vi "StartMods.vi"(7 "ShowPanel? (f)":bool=TRUE, 8 "ErrorArray":errorcluster[](array[cluster]), 10 "ModuleList":string[](array[string]), 11 "Test.lvclass":refnum<class "Test.lvclass">) -> (0 "ErrorArray":errorcluster[](array[cluster]), 2 "Events":variant[](array[variant]), 3 "Test.lvclass":refnum<class "Test.lvclass">)   [LabVIEW 2018, in "Test.lvclass"]
doc: "This VI instantiates a module..."
uses:
  Test.lvclass
  <userlib>/NIST/ModuleAdminLib/ModuleAdmin/ModuleAdmin.lvclass/ModuleAdmin.ctl
  <userlib>/NIST/ModuleAdminLib/CloneRegistration/CloneRegistration.lvclass
  Test.lvclass/Test.ctl
  <userlib>/NIST/ModuleAdminLib/ModuleAdmin/Accessors/Read CloneRegRef.vi
  Accessors/Write ModuleList.vi
  Accessors/Write ModuleIDs.vi
  Accessors/Write CloneReg.vi
  <vilib>/Utility/error.llb/Error Cluster From Error Code.vi
  <vilib>/ErrorRing/Error Ring.xnode
  <userlib>/NIST/ModuleAdminLib/ModuleAdmin/ModuleAdmin.lvclass
  <userlib>/NIST/NISTErrorLib/NISTErrorLib.lvlib
  Sync/SyncModule/SyncModule.lvlib
  Digitizer/DigitizerModule/DigitizerModule.lvlib
  FGen/FgenModule/FgenModule.lvlib
  Analysis/AnalysisModule/AnalysisModule.lvlib
  Sensor/SensorModule/SensorModule.lvlib
  Scope/ScopeModule/ScopeModule.lvlib
  AcPwr/AcPwrModule/AcPwrModule.lvlib
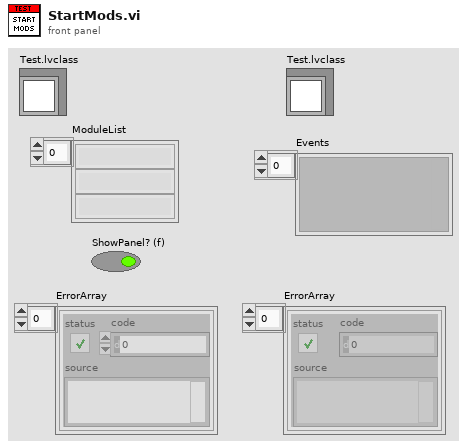
[diagram p1: front panel]
types:
  T1 = typedef "SyncModule.lvlib/clBroadcastEvents.ctl" = cluster{"DidInit":refnum<user-event>, "StatusUpdate":refnum<user-event>, "ErrorReport":refnum<user-event>, "DidStop":refnum<user-event>, "PathToINI":refnum<user-event>, "TriggerTime":refnum<user-event>, "LockStatus":refnum<user-event>, "Info":refnum<user-event>}
  T2 = typedef "FgenModule.lvlib/clBroadcastEvents.ctl" = cluster{"DidInit":refnum<user-event>, "StatusUpdate":refnum<user-event>, "ErrorReport":refnum<user-event>, "DidStop":refnum<user-event>, "PathToINI":refnum<user-event>, "Channels":refnum<user-event>, "Function":refnum<user-event>, "Waveforms":refnum<user-event>, "Triggers":refnum<user-event>, "FunctionParams":refnum<user-event>}
  T3 = typedef "DigitizerModule.lvlib/clBroadcastEvents.ctl" = cluster{"DidInit":refnum<user-event>, "StatusUpdate":refnum<user-event>, "ErrorReport":refnum<user-event>, "DidStop":refnum<user-event>, "PathToINI":refnum<user-event>, "Channels":refnum<user-event>, "Acq":refnum<user-event>, "Trigger":refnum<user-event>, "Waveforms":refnum<user-event>}
  T4 = typedef "ScopeModule.lvlib/clBroadcastEvents.ctl" = cluster{"DidInit":refnum<user-event>, "StatusUpdate":refnum<user-event>, "ErrorReport":refnum<user-event>, "DidStop":refnum<user-event>, "PathToINI":refnum<user-event>, "Handle":refnum<user-event>, "Model":refnum<user-event>, "Channels":refnum<user-event>, "Acquisition":refnum<user-event>, "Trigger":refnum<user-event>, "ExtAcquisition":refnum<user-event>, "Waveform":refnum<user-event>}
  T5 = typedef "SensorModule.lvlib/clBroadcastEvents.ctl" = cluster{"DidInit":refnum<user-event>, "StatusUpdate":refnum<user-event>, "ErrorReport":refnum<user-event>, "DidStop":refnum<user-event>, "PathToINI":refnum<user-event>, "SensorReport":refnum<user-event>, "SensorConfig":refnum<user-event>}
  T6 = typedef "AnalysisModule.lvlib/clBroadcastEvents.ctl" = cluster{"DidInit":refnum<user-event>, "StatusUpdate":refnum<user-event>, "ErrorReport":refnum<user-event>, "DidStop":refnum<user-event>, "PathToINI":refnum<user-event>, "Config":refnum<user-event>, "ResultReport":refnum<user-event>, "FunctionClass":refnum<user-event>}
  T7 = typedef "AcPwrModule.lvlib/clBroadcastEvents.ctl" = cluster{"DidInit":refnum<user-event>, "StatusUpdate":refnum<user-event>, "ErrorReport":refnum<user-event>, "DidStop":refnum<user-event>, "PathToINI":refnum<user-event>, "Measurements":refnum<user-event>, "LoadConfigFile":refnum<user-event>, "GetSettings":refnum<user-event>, "SetSettings":refnum<user-event>, "GetType&ID":refnum<user-event>, "GotSettings":refnum<user-event>}
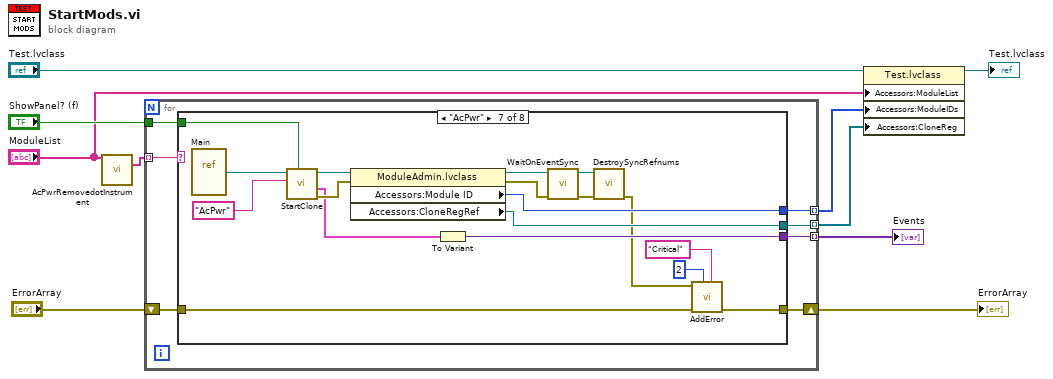
[diagram p0: block diagram]
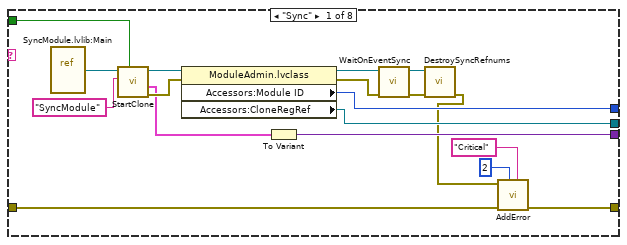
[diagram p2: hidden frame]
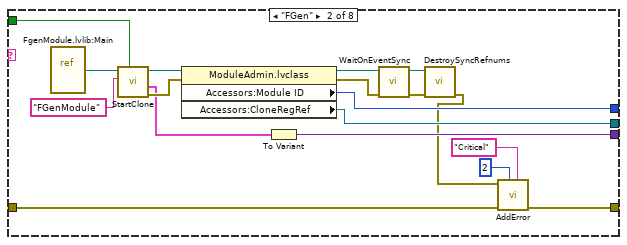
[diagram p3: hidden frame]
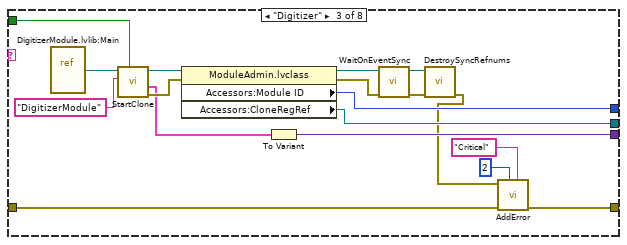
[diagram p4: hidden frame]
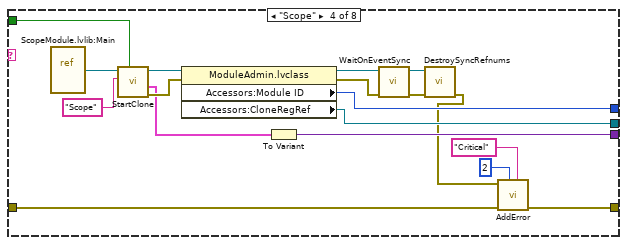
[diagram p5: hidden frame]
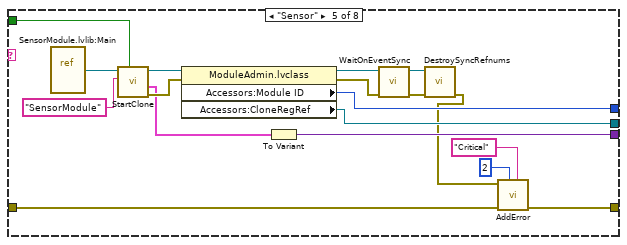
[diagram p6: hidden frame]
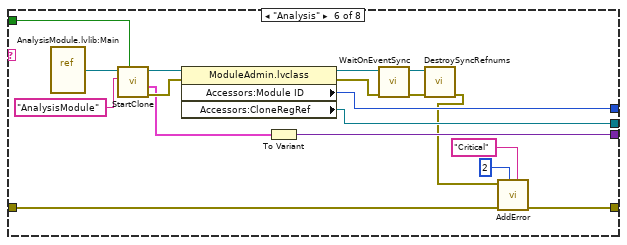
[diagram p7: hidden frame]
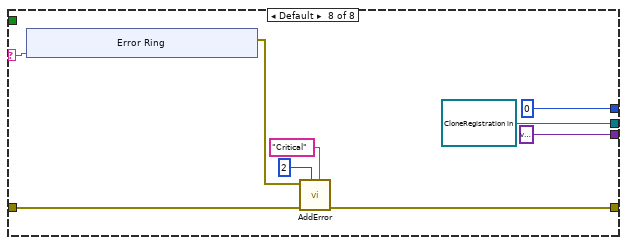
[diagram p8: hidden frame]
diagram:
  n1 = call "AcPwrRemovedotInstrument.vi"("ModuleListArray"="ModuleList") -> ("BeforeMatch:ModuleListArray"=w1:string[])  [unwired: 10 in, 4 out]
  n2 = for {
    tunnel: w1 -> [w11] mode=indexing
    shift-right: [w16] -> w6
    shift-left: "ErrorArray" -> [w17]
    tunnel: [w15] -> w9 mode=indexing
    tunnel: [w14] -> w7 mode=indexing
    tunnel: [w13] -> w5 mode=indexing
    tunnel: "ShowPanel? (f)" -> [w12]
    n3 = case shown="\"AcPwr\"" w11 {
      selector: w11 -> [_ _ _ _ _ _ _ w152]
      tunnel: w17 -> [w20 w38 w56 w74 w92 w110 w129 w151]
      tunnel: [w23 w41 w59 w77 w95 w113 w132 w147] -> w16
      tunnel: [w24 w42 w60 w78 w96 w114 w133 variant ("Variant")] -> w15
      tunnel: [w26 w44 w62 w80 w98 w116 w135 refnum<data-value> refnum ("Accessors:CloneRegRef")] -> w14
      tunnel: [w25 w43 w61 w79 w97 w115 w134 0 ("Accessors:Module ID")] -> w13
      tunnel: w12 -> [w18 w36 w54 w72 w90 w108 w127 _]
      frame "Sync" {
        n4 = vi-ref "SyncModule.lvlib:Main.vi"() -> (w35:refnum<vi>)
        n5 = call "StartClone.vi"("ShowPanel? (f)"=w18, "ModuleName"="SyncModule", "VI Refnum"=w35) -> ("error out"=w28:errorcluster, "SyncBroadcastEvents"=w27:T1, "ModuleAdmin"=w33:refnum<class "ModuleAdmin.lvclass">)  [unwired: 6 in]
        n6 = property class="ModuleAdmin.lvclass"(reference=w33, error in=w28) -> (reference out=w31:refnum<class "ModuleAdmin.lvclass">, error out=w32:errorcluster, "Accessors:Module ID"=w25:i32, "Accessors:CloneRegRef"=w26:refnum<data-value>)
        n7 = To Variant(anything=w27) -> (Variant=w24:variant)
        n8 = call <userlib>:"WaitOnEventSync.vi"("error in (no error)"=w32, "ModuleAdmin"=w31) -> ("error out"=w30:errorcluster, "ModuleAdmin"=w29:refnum<class "ModuleAdmin.lvclass">)  [unwired: 8 in]
        n9 = call <userlib>:"DestroySyncRefnums.vi"("error in (no error)"=w30, "ModuleAdmin"=w29) -> ("error out"=w19:errorcluster)  [unwired: 9 in]
        n10 = call <userlib>:"AddError.vi"("Severity"="Critical", "Priority"=u8 2, "ErrorArray"=w20, "error in (no error)"=w19) -> ("ErrorArray"=w23:errorcluster[])  [unwired: 6 in, 1 out]
      }
      frame "FGen" {
        n11 = vi-ref "FgenModule.lvlib:Main.vi"() -> (w53:refnum<vi>)
        n12 = call "StartClone.vi"("ShowPanel? (f)"=w36, "ModuleName"="FGenModule", "VI Refnum"=w53) -> ("error out"=w46:errorcluster, "clBroadcastEvents"=w45:T2, "ModuleAdmin"=w51:refnum<class "ModuleAdmin.lvclass">)  [unwired: 6 in]
        n13 = property class="ModuleAdmin.lvclass"(reference=w51, error in=w46) -> (reference out=w49:refnum<class "ModuleAdmin.lvclass">, error out=w50:errorcluster, "Accessors:Module ID"=w43:i32, "Accessors:CloneRegRef"=w44:refnum<data-value>)
        n14 = To Variant(anything=w45) -> (Variant=w42:variant)
        n15 = call <userlib>:"WaitOnEventSync.vi"("error in (no error)"=w50, "ModuleAdmin"=w49) -> ("error out"=w48:errorcluster, "ModuleAdmin"=w47:refnum<class "ModuleAdmin.lvclass">)  [unwired: 8 in]
        n16 = call <userlib>:"DestroySyncRefnums.vi"("error in (no error)"=w48, "ModuleAdmin"=w47) -> ("error out"=w37:errorcluster)  [unwired: 9 in]
        n17 = call <userlib>:"AddError.vi"("Severity"="Critical", "Priority"=u8 2, "ErrorArray"=w38, "error in (no error)"=w37) -> ("ErrorArray"=w41:errorcluster[])  [unwired: 6 in, 1 out]
      }
      frame "Digitizer" {
        n18 = vi-ref "DigitizerModule.lvlib:Main.vi"() -> (w71:refnum<vi>)
        n19 = call "StartClone.vi"("ShowPanel? (f)"=w54, "ModuleName"="DigitizerModule", "VI Refnum"=w71) -> ("error out"=w64:errorcluster, "clBroadcastEvents"=w63:T3, "ModuleAdmin"=w69:refnum<class "ModuleAdmin.lvclass">)  [unwired: 6 in]
        n20 = property class="ModuleAdmin.lvclass"(reference=w69, error in=w64) -> (reference out=w67:refnum<class "ModuleAdmin.lvclass">, error out=w68:errorcluster, "Accessors:Module ID"=w61:i32, "Accessors:CloneRegRef"=w62:refnum<data-value>)
        n21 = To Variant(anything=w63) -> (Variant=w60:variant)
        n22 = call <userlib>:"WaitOnEventSync.vi"("error in (no error)"=w68, "ModuleAdmin"=w67) -> ("error out"=w66:errorcluster, "ModuleAdmin"=w65:refnum<class "ModuleAdmin.lvclass">)  [unwired: 8 in]
        n23 = call <userlib>:"DestroySyncRefnums.vi"("error in (no error)"=w66, "ModuleAdmin"=w65) -> ("error out"=w55:errorcluster)  [unwired: 9 in]
        n24 = call <userlib>:"AddError.vi"("Severity"="Critical", "Priority"=u8 2, "ErrorArray"=w56, "error in (no error)"=w55) -> ("ErrorArray"=w59:errorcluster[])  [unwired: 6 in, 1 out]
      }
      frame "Scope" {
        n25 = vi-ref "ScopeModule.lvlib:Main.vi"() -> (w89:refnum<vi>)
        n26 = call "StartClone.vi"("ShowPanel? (f)"=w72, "ModuleName"="Scope", "VI Refnum"=w89) -> ("error out"=w82:errorcluster, "clBroadcastEvents"=w81:T4, "ModuleAdmin"=w87:refnum<class "ModuleAdmin.lvclass">)  [unwired: 6 in]
        n27 = property class="ModuleAdmin.lvclass"(reference=w87, error in=w82) -> (reference out=w85:refnum<class "ModuleAdmin.lvclass">, error out=w86:errorcluster, "Accessors:Module ID"=w79:i32, "Accessors:CloneRegRef"=w80:refnum<data-value>)
        n28 = To Variant(anything=w81) -> (Variant=w78:variant)
        n29 = call <userlib>:"WaitOnEventSync.vi"("error in (no error)"=w86, "ModuleAdmin"=w85) -> ("error out"=w84:errorcluster, "ModuleAdmin"=w83:refnum<class "ModuleAdmin.lvclass">)  [unwired: 8 in]
        n30 = call <userlib>:"DestroySyncRefnums.vi"("error in (no error)"=w84, "ModuleAdmin"=w83) -> ("error out"=w73:errorcluster)  [unwired: 9 in]
        n31 = call <userlib>:"AddError.vi"("Severity"="Critical", "Priority"=u8 2, "ErrorArray"=w74, "error in (no error)"=w73) -> ("ErrorArray"=w77:errorcluster[])  [unwired: 6 in, 1 out]
      }
      frame "Sensor" {
        n32 = vi-ref "SensorModule.lvlib:Main.vi"() -> (w107:refnum<vi>)
        n33 = call "StartClone.vi"("ShowPanel? (f)"=w90, "ModuleName"="SensorModule", "VI Refnum"=w107) -> ("error out"=w100:errorcluster, "clBroadcastEvents"=w99:T5, "ModuleAdmin"=w105:refnum<class "ModuleAdmin.lvclass">)  [unwired: 6 in]
        n34 = property class="ModuleAdmin.lvclass"(reference=w105, error in=w100) -> (reference out=w103:refnum<class "ModuleAdmin.lvclass">, error out=w104:errorcluster, "Accessors:Module ID"=w97:i32, "Accessors:CloneRegRef"=w98:refnum<data-value>)
        n35 = To Variant(anything=w99) -> (Variant=w96:variant)
        n36 = call <userlib>:"WaitOnEventSync.vi"("error in (no error)"=w104, "ModuleAdmin"=w103) -> ("error out"=w102:errorcluster, "ModuleAdmin"=w101:refnum<class "ModuleAdmin.lvclass">)  [unwired: 8 in]
        n37 = call <userlib>:"DestroySyncRefnums.vi"("error in (no error)"=w102, "ModuleAdmin"=w101) -> ("error out"=w91:errorcluster)  [unwired: 9 in]
        n38 = call <userlib>:"AddError.vi"("Severity"="Critical", "Priority"=u8 2, "ErrorArray"=w92, "error in (no error)"=w91) -> ("ErrorArray"=w95:errorcluster[])  [unwired: 6 in, 1 out]
      }
      frame "Analysis" {
        n39 = vi-ref "AnalysisModule.lvlib:Main.vi"() -> (w125:refnum<vi>)
        n40 = call "StartClone.vi"("ShowPanel? (f)"=w108, "ModuleName"="AnalysisModule", "VI Refnum"=w125) -> ("error out"=w118:errorcluster, "AnalysisBroadcastEvents"=w117:T6, "ModuleAdmin"=w123:refnum<class "ModuleAdmin.lvclass">)  [unwired: 6 in]
        n41 = property class="ModuleAdmin.lvclass"(reference=w123, error in=w118) -> (reference out=w121:refnum<class "ModuleAdmin.lvclass">, error out=w122:errorcluster, "Accessors:Module ID"=w115:i32, "Accessors:CloneRegRef"=w116:refnum<data-value>)
        n42 = To Variant(anything=w117) -> (Variant=w114:variant)
        n43 = call <userlib>:"WaitOnEventSync.vi"("error in (no error)"=w122, "ModuleAdmin"=w121) -> ("error out"=w120:errorcluster, "ModuleAdmin"=w119:refnum<class "ModuleAdmin.lvclass">)  [unwired: 8 in]
        n44 = call <userlib>:"DestroySyncRefnums.vi"("error in (no error)"=w120, "ModuleAdmin"=w119) -> ("error out"=w109:errorcluster)  [unwired: 9 in]
        n45 = call <userlib>:"AddError.vi"("Severity"="Critical", "Priority"=u8 2, "ErrorArray"=w110, "error in (no error)"=w109) -> ("ErrorArray"=w113:errorcluster[])  [unwired: 6 in, 1 out]
      }
      frame "AcPwr" {
        n46 = vi-ref "Main.vi"() -> (w126:refnum<vi>)
        n47 = call "StartClone.vi"("ShowPanel? (f)"=w127, "ModuleName"="AcPwr", "VI Refnum"=w126) -> ("error out"=w137:errorcluster, "clBroadcastEvents"=w136:T7, "ModuleAdmin"=w142:refnum<class "ModuleAdmin.lvclass">)  [unwired: 6 in]
        n48 = property class="ModuleAdmin.lvclass"(reference=w142, error in=w137) -> (reference out=w140:refnum<class "ModuleAdmin.lvclass">, error out=w141:errorcluster, "Accessors:Module ID"=w134:i32, "Accessors:CloneRegRef"=w135:refnum<data-value>)
        n49 = To Variant(anything=w136) -> (Variant=w133:variant)
        n50 = call <userlib>:"WaitOnEventSync.vi"("error in (no error)"=w141, "ModuleAdmin"=w140) -> ("error out"=w139:errorcluster, "ModuleAdmin"=w138:refnum<class "ModuleAdmin.lvclass">)  [unwired: 8 in]
        n51 = call <userlib>:"DestroySyncRefnums.vi"("error in (no error)"=w139, "ModuleAdmin"=w138) -> ("error out"=w128:errorcluster)  [unwired: 9 in]
        n52 = call <userlib>:"AddError.vi"("Severity"="Critical", "Priority"=u8 2, "ErrorArray"=w129, "error in (no error)"=w128) -> ("ErrorArray"=w132:errorcluster[])  [unwired: 6 in, 1 out]
      }
      frame Default {
        n53 = xnode "Error Ring"("parameter 0"=w152) -> ("error out"=w150:errorcluster)
        n54 = call <userlib>:"AddError.vi"("Severity"="Critical", "Priority"=u8 2, "ErrorArray"=w151, "error in (no error)"=w150) -> ("ErrorArray"=w147:errorcluster[])  [unwired: 6 in, 1 out]
      }
    }
  }
  "ErrorArray" <- w6
  "Events" <- w9
  n55 = property class="Test.lvclass"(reference="Test.lvclass", "Accessors:ModuleList"="ModuleList", "Accessors:ModuleIDs"=w5, "Accessors:CloneReg"=w7) -> (reference out=→"Test.lvclass":refnum<class "Test.lvclass">)  [unwired: 1 in, 1 out]
